vi "TopicRequest_Respond.vi"(3 "port":u16, 4 "XML":string) -> (1 "Topic Request Reply":string, 2 "New Subscriber":T1)   [LabVIEW 2012]
doc: "Builds the reply to the \"requestTopic\" Slave API method. Also returns a ROS reference to the new subscriber.\n\nCurrently only supports the TCPROS protocol."
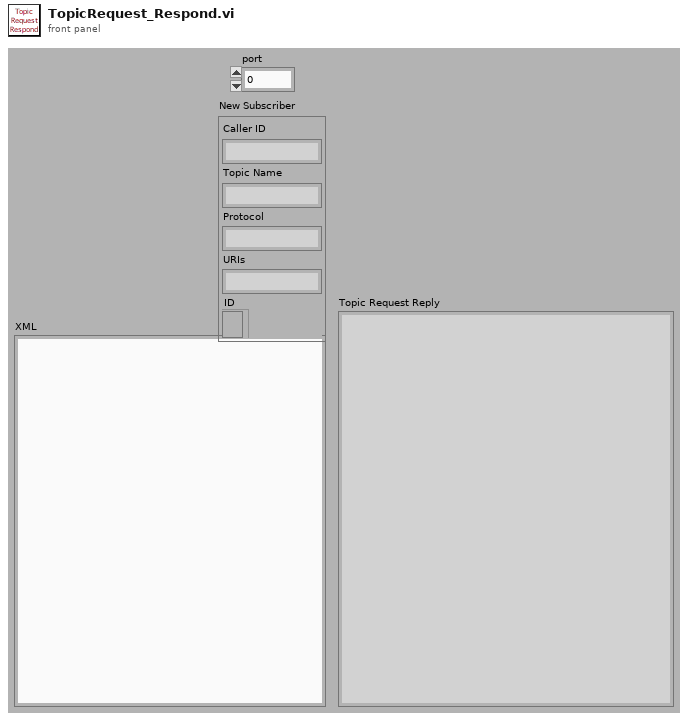
[diagram p1: front panel]
types:
  T1 = cluster{"Caller ID":string, "Topic Name":string, "Protocol":string, "URIs":string, "ID":refnum<k5>}
  T2 = enum16{"http://IP:port", "http://IP", "IP:port", "IP only"}
  T3 = cluster{"Caller ID":string, "Topic Name":string, "Protocol":string, "URI":string, "ID":refnum<k5>}
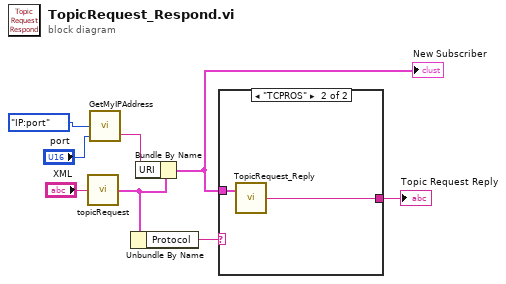
[diagram p0: block diagram]
diagram:
  n1 = call "topicRequest.vi"("XML"="XML") -> ("Subscriber"=w5:T3)
  n2 = call "GetMyIPAddress.vi"("Port"="port", "Format"=T2."IP:port") -> ("URI"=w2:string)  [unwired: 2 in]
  n3 = Unbundle By Name(w5) -> ("Protocol"=w7:string)
  n4 = Bundle By Name(cluster=w5, "URI"=w2) -> (w1:T3)
  "New Subscriber" <- w1
  n5 = case shown="\"TCPROS\"" w7 {
    tunnel: w1 -> [_ w9]
    tunnel: [_ w10] -> w6
    frame Default {
    }
    frame "TCPROS" {
      n6 = call "TopicRequest_Reply.vi"("Subscriber"=w9) -> ("XML"=w10:string)  [unwired: 1 in]
    }
  }
  "Topic Request Reply" <- w6
